vi "programa_main.vi"() -> ()   [LabVIEW 2017]
uses:
  ble_toolkit_source/type_def/connection_status_bundle.ctl
  ble_toolkit_source/type_def/address_type.ctl
  <vilib>/Platform/TimedLoop/XDataNode/timing_clust.ctl
  <vilib>/Platform/TimedLoop/XDataNode/nitl_modes.ctl
  <vilib>/Platform/TimedLoop/XDataNode/wakeup.ctl
  <vilib>/Instr/_visa.llb/VISA Configure Serial Port (Instr).vi
  <vilib>/platform/TimedLoop/XDataNode/XDataNode.xnode
  <vilib>/Platform/TimedLoop/XDataNode/XDNodeRunTimeDep.lvlib
panel:
  out "Energia consumida (mA·h)":dbl
  in  "Automàtic":bool
  in  "Manual":bool
  out "READY":bool
  in  "No Rebre Corrent":bool
  in  "Rebre Corrent":bool
  in  "No Rebre Voltatge Placa":bool
  in  "Rebre Placa":bool
  in  "No Rebre Posició":bool
  in  "Rebre Posició":bool
  in  "VISA resource name":refnum<visa-resource-name>="COM1"
  out "MAC Adrdress Seleccionada":string
  in  "MAC Address":T1=1 items=["Rueda", "Nelia"]
  out "Nom del dispsitiu conectat":string
  out "Handle table 2":string[][](array[string])
  out "Scanning":bool
  in  "Address Type":T1=1 items=["Public", "Random"]
  in  "COM Bluegiga in":refnum<visa-resource-name>="COM13"
  out "Devices":string[][](array[string])
  out "BLED112 Dongle Info":string
  out "nom fitxer":string
  out "Lectura":string
  out "Posició (º)":dbl
  out "Intensitat (mA)":dbl
  in  "?":bool
  out "Waveform Chart":dynamicdata(graph)
  out "Volatatge (V)":dbl
  out "Connection Status":T2={"MAC Address"="", "cnx handle"=0, "cnx flags"=0, "Address Type"=125, "Connection Interval (ms)"=125, "Timeout(ms)"=125, "Latency"=0, "bonding handle"=0} {"Address Type" items=["Public", "Random"]}
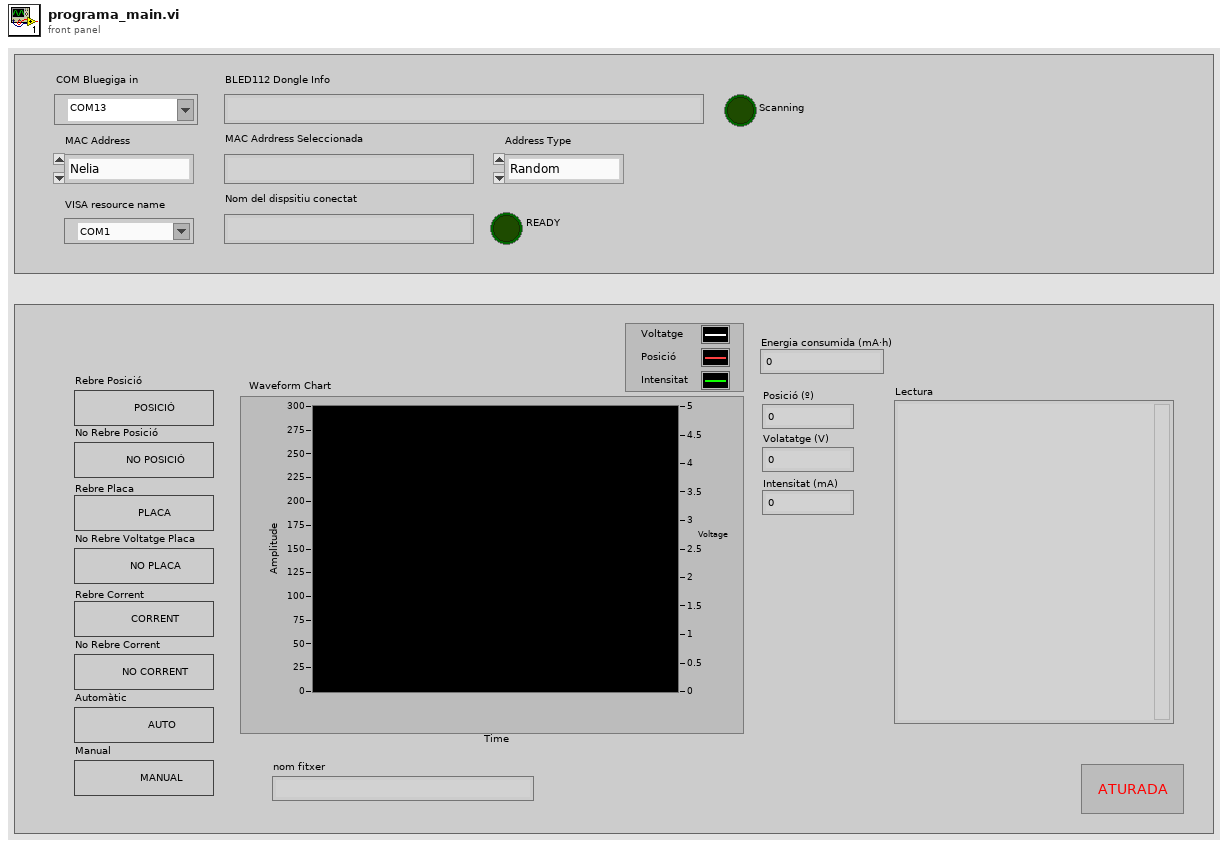
[diagram p1: front panel]
types:
  T1 = typedef "address_type.ctl" = u8
  T2 = typedef "connection_status_bundle.ctl" = cluster{"MAC Address":string, "cnx handle":u8, "cnx flags":u8, "Address Type":T1, "Connection Interval (ms)":u16, "Timeout(ms)":u16, "Latency":u16, "bonding handle":u8}
  T3 = typedef "XDNodeRunTimeDep.lvlib/timing_clust.ctl" = cluster{"Expected End [f-1]":u64, "Actual End [f-1]":u64, "Finished Late? [f-1]":bool, "Expected End [i-1]":u64, "Actual End [i-1]":u64, "Finished Late? [i-1]":bool, "Expected Start [i]":u64, "Actual Start [i]":u64, "Expected Start [f]":u64, "Actual Start [f]":u64, "Source Name":string, "Structure Name":string, "Period":i64, "Deadline":i64, "Offset":i64, "Start":i64, "Priority":i32, "Timeout":i32, "Mode":T4, "Wakeup Reason":T5, "Error":errorcluster, "Source Type":string, "Secondary Source Type":string, "Global End Time":u64, "Global Start Time":u64, "Frame Duration":u64, "Iteration Duration":u64, "Assigned CPU":i32, "I/O Scan Engine Mode":u32}
  T4 = typedef "XDNodeRunTimeDep.lvlib/nitl_modes.ctl" = enum32{"No Change", "Process missed periods, maintain original phase", "Discard missed periods, maintain original phase", "Process missed periods, ignore original phase", "Discard missed periods, ignore original phase"}
  T5 = typedef "XDNodeRunTimeDep.lvlib/wakeup.ctl" = enum32{"Normal", "Aborted", "Asynchronous wakeup", "Timing source error", "Timed loop error", "Timeout"}
  T6 = typedef "LVDateTimeRec.ctl" = cluster{"fractional second":dbl, "second":i32, "minute":i32, "hour":i32, "day of month":i32, "month":i32, "year":i32, "day of week":i32, "day of year":i32, "DST":i32}
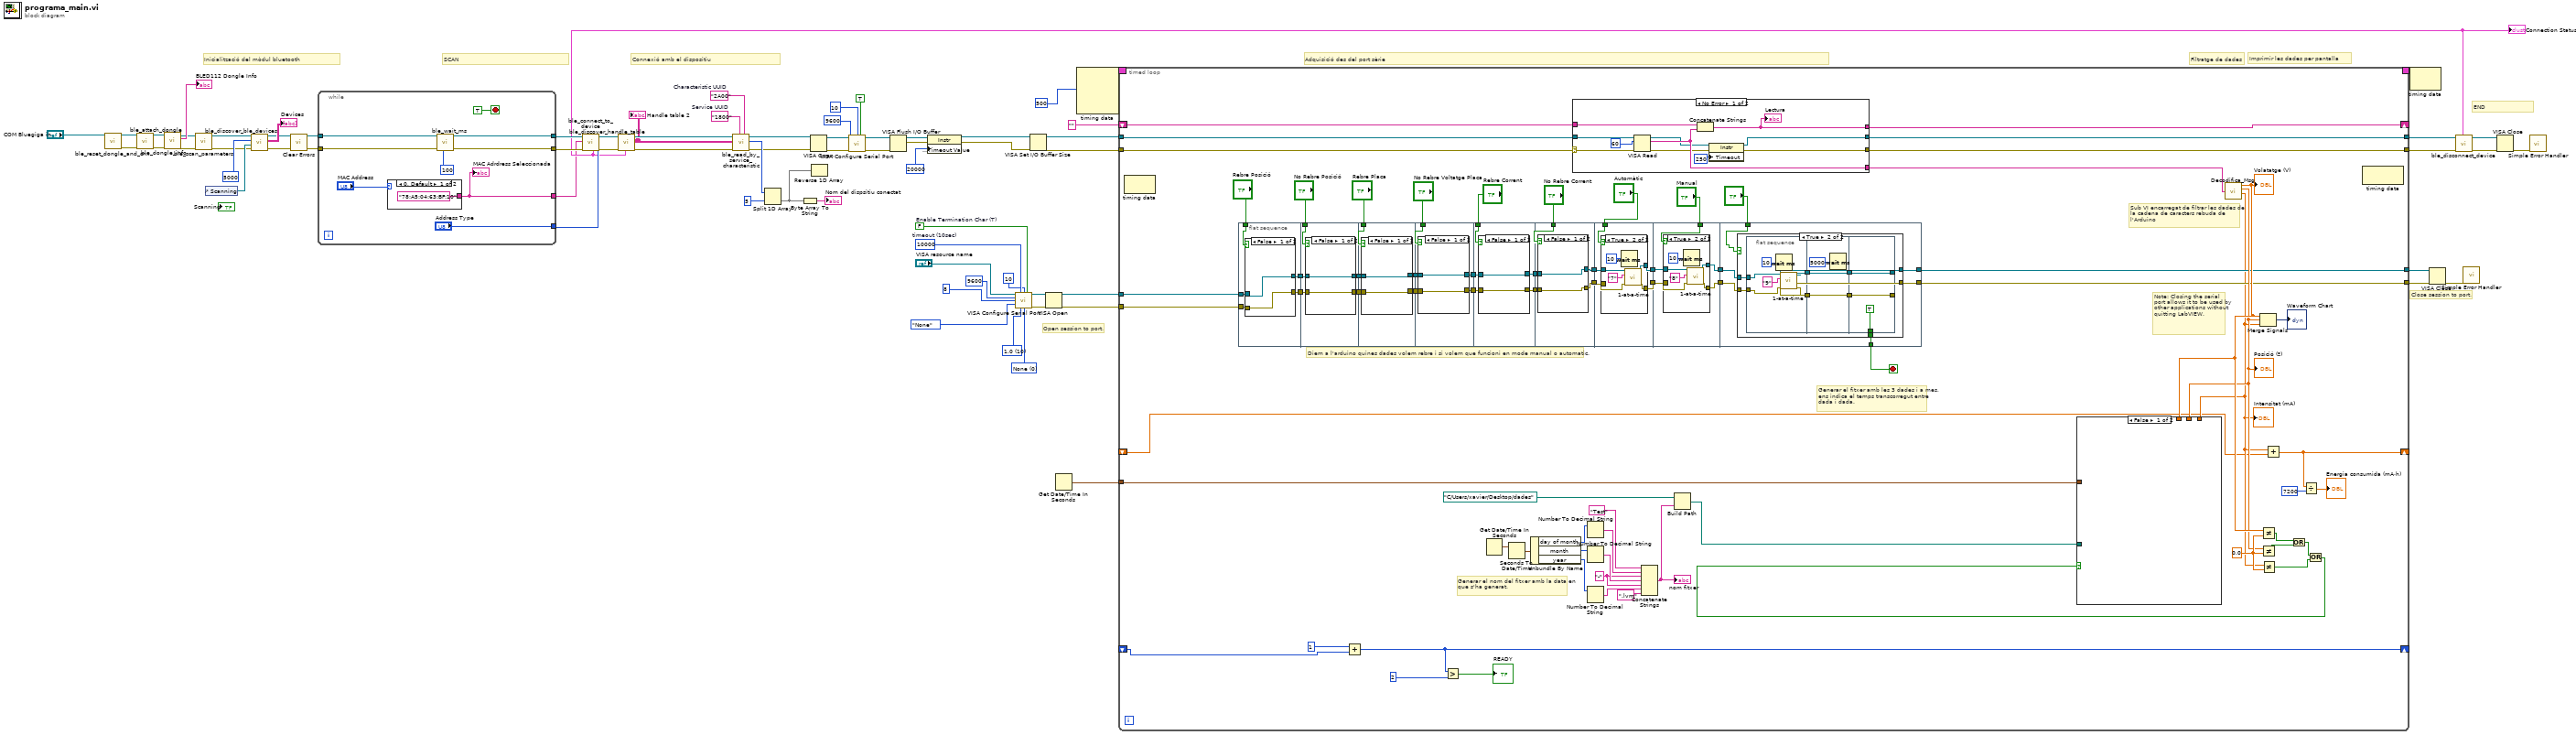
[diagram p0: block diagram]
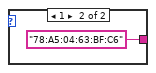
[diagram p2: hidden frame]
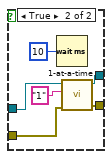
[diagram p3: hidden frame]
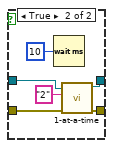
[diagram p4: hidden frame]
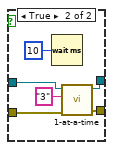
[diagram p5: hidden frame]
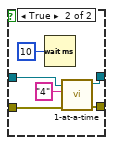
[diagram p6: hidden frame]
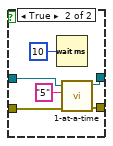
[diagram p7: hidden frame]
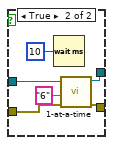
[diagram p8: hidden frame]
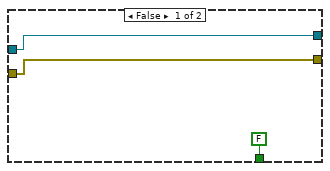
[diagram p11: hidden frame]
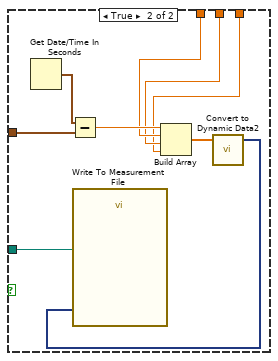
[diagram p12: hidden frame]
diagram:
  w5 = u16 0 items=["None", "XON/XOFF", "RTS/CTS", "XON/XOFF & RTS/CTS", "DTR/DSR", "XON/XOFF & DTR/DSR"] ("flow control (0:none)")
  w6 = u16 10 items=["1.0"=10, "1.5"=15, "2.0"=20] ("stop bits (10: 1 bit)")
  w17 = FALSE  # Enable Termination Char (T)
  w16 = u32 10000  # timeout (10sec)
  w32 = "2A00"  # Characteristic UUID
  w33 = "1800"  # Service UUID
  # "Open session to port."
  # "Close session to port."
  # "Imprimir les dades per pantalla"
  # "Filtratge de dades"
  # "Adquisició des del port sèrie"
  # "Connexió amb el dispositiu"
  # "SCAN"
  # "END"
  # "Inicialització del mòdul bluetooth"
  n1 = call "ble_reset_dongle_and_cnx.vi"("COM Bluegiga in"="COM Bluegiga in") -> ("error out"=w51:errorcluster, "COM Bluegiga out"=w49:refnum<visa-resource-name>)  [unwired: 9 in]
  n2 = call "ble_attach_dongle.vi"("error in (no error)"=w51, "COM Bluegiga in"=w49) -> ("error out"=w53:errorcluster, "COM Bluegiga out"=w52:refnum<visa-resource-name>)  [unwired: 8 in]
  n3 = call "ble_dongle_info.vi"("error in (no error)"=w53, "COM Bluegiga in"=w52) -> ("error out"=w56:errorcluster, "info"=→"BLED112 Dongle Info":string, "COM Bluegiga out"=w57:refnum<visa-resource-name>)  [unwired: 7 in]
  n4 = call "ble_scan_parameters.vi"("error in (no error)"=w56, "COM Bluegiga in"=w57) -> ("error out"=w54:errorcluster, "COM Bluegiga out"=w55:refnum<visa-resource-name>)  [unwired: 7 in, 1 out]
  n5 = control-ref of="Scanning"() -> (w60:refnum<vi>)
  n6 = call "ble_discover_ble_devices.vi"("error in (no error)"=w54, "LED ref"=w60, "Scan Duration (10000ms)"=u32 5000, "COM Bluegiga in"=w55) -> ("error out"=w48:errorcluster, "Devices"=→"Devices":string[][], "COM Bluegiga out"=w61:refnum<visa-resource-name>)  [unwired: 5 in]
  n7 = call <vilib>:"Clear Errors.vi"("error in (no error)"=w48) -> ("error out"=w47:errorcluster)  [unwired: 5 in, 1 out]
  n8 = while {
    tunnel: w47 -> [w82]
    tunnel: [w81] -> w59
    tunnel: w61 -> [w81]
    tunnel: [w80] -> w58
    tunnel: ["Address Type"] -> w46
    tunnel: [w76] -> w21
    stop <- TRUE stop-if-true
    n9 = case shown="0, Default" "MAC Address" {
      tunnel: ["78:A5:04:63:BF:10" "78:A5:04:63:BF:C6"] -> w76
      frame 0, Default {
      }
      frame 1 {
      }
    }
    "MAC Adrdress Seleccionada" <- w76
    n10 = call "ble_wait_ms.vi"("milliseconds to wait (100)"=u32 100, "error in (no error)"=w82) -> ("error out"=w80:errorcluster)  [unwired: 9 in]
  }
  n11 = call "ble_connect_to_device.vi"("Address Type"=w46, "error in (no error)"=w58, "MAC Address"=w21, "COM Bluegiga in"=w59) -> ("error out"=w27:errorcluster, "COM Bluegiga out"=w28:refnum<visa-resource-name>, "Connection Status"=w22:T2)  [unwired: 5 in]
  "Connection Status" <- w22
  n12 = call "ble_discover_handle_table.vi"("Connection Status"=w22, "error in (no error)"=w27, "COM Bluegiga in"=w28) -> ("error out"=w37:errorcluster, "Handle table"=w31:string[][], "COM Bluegiga out"=w36:refnum<visa-resource-name>)  [unwired: 6 in]
  "Handle table 2" <- w31
  n13 = call "ble_read_by_service_characteristic.vi"("Characteristic UUID"=w32, "Service UUID"=w33, "error in (no error)"=w37, "Handle table"=w31, "COM Bluegiga in"=w36) -> ("error out"=w25:errorcluster, "characteristic value"=w30:u8[], "COM Bluegiga out"=w26:refnum<visa-resource-name>)  [unwired: 4 in]
  n14 = Split 1D Array(array=w30, index=5) -> (second subarray=w29:u8[])  [unwired: 1 out]
  n15 = Byte Array To String(unsigned byte array=w29) -> (string=→"Nom del dispsitiu conectat":string)
  n16 = VISA Open(error in (no error)=w25, VISA resource name=w26) -> (VISA resource name=w45:refnum<visa-resource-name>, error out=w24:errorcluster)  [unwired: 3 in]
  n17 = Reverse 1D Array(array=w29) -> ()  [unwired: 1 out]
  n18 = call-poly "VISA Configure Serial Port"("VISA resource name"=w45, "termination char\n(0xA = '\\n' = LF)"=u8 10 ("termination char\n(0xA = '\\n' = LF)"), "Enable Termination\nChar (T)"=TRUE ("Enable Termination\nChar (T)"), "baud rate (9600)"=u32 9600, "error in (no error)"=w24) -> ("VISA resource name out"=w42:refnum<visa-resource-name>, "error out"=w23:errorcluster)  [unwired: 9 in]
  n19 = VISA Flush I/O Buffer(VISA resource name=w42, error in (no error)=w23) -> (VISA resource name out=w40:refnum<visa-resource-name>, error out=w39:errorcluster)  [unwired: 1 in]
  n20 = property class="Instr"(reference=w40, error in=w39, "General Settings:Timeout Value"=u32 20000) -> (reference out=w2:refnum<visa-resource-name>, error out=w1:errorcluster)
  n21 = call-poly "VISA Configure Serial Port"("VISA resource name"="VISA resource name", "timeout (10sec)"=w16, "termination char\n(0xA = '\\n' = LF)"=u8 10 ("termination char\n(0xA = '\\n' = LF)"), "Enable Termination\nChar (T)"=w17, "baud rate (9600)"=u32 9600, "data bits (8)"=u16 8, "parity (0:none)"=enum16{"None", "Odd", "Even", "Mark", "Space"}."None", "stop bits (10: 1 bit)"=w6, "flow control (0:none)"=w5) -> ("VISA resource name out"=w18:refnum<visa-resource-name>, "error out"=w19:errorcluster)  [unwired: 5 in]
  n22 = VISA Set I/O Buffer Size(VISA resource name=w2, error in (no error)=w1) -> (VISA resource name out=w4:refnum<visa-resource-name>, error out=w3:errorcluster)  [unwired: 2 in]
  n23 = VISA Open(error in (no error)=w19, VISA resource name=w18) -> (VISA resource name=w14:refnum<visa-resource-name>, error out=w13:errorcluster)  [unwired: 3 in]
  n24 = Get Date/Time In Seconds() -> (seconds since 1Jan1904=w65:timestamp)
  n25 = node-c288(i64 500 ("Period")) -> (w68:T3)  [unwired: 3 in]
  n26 = timed-loop {
    tunnel: w4 -> [w125]
    tunnel: w3 -> [w126]
    shift-right: [w153] -> _
    shift-left: "" ("read buffer") -> [w155]
    tunnel: [w152] -> w69
    tunnel: [w151] -> w70
    timing: w68 -> [_]
    timing-out: [_] -> w67
    tunnel: w65 -> [w129]
    tunnel: w14 -> [w118]
    tunnel: w13 -> [w105]
    tunnel: [w112] -> w12
    tunnel: [w111] -> w11
    shift-right: [w102] -> _
    shift-left: _ -> [w103]
    shift-right: [w89] -> _
    shift-left: _ -> [w92]
    stop <- w85 stop-if-true
    w130 = 0.0
    w142 = "-" ("string")
    # "Diem a l'arduino quines dades volem rebre i si volem que funcioni en mode manual o automatic."
    # "Generar el fitxer amb les 3 dades i a mes, ens indica el temps transcorregut entre dada i dada."
    # "Generar el nom del fitxer amb la data en que s'ha generat."
    # "Sub VI encarregat de filtrar les dades de la cadena de caracters rebuda de l'Arduino"
    # "Note: Closing the serial port allows it to be used by other applications without\nquitting LabVIEW."
    n27 = node-c288() -> ()  [unwired: 1 in, 1 out]
    n28 = flat-sequence {
      tunnel: "Rebre Posició" -> [w160]
      tunnel: w118 -> [w159]
      tunnel: [w158] -> w117
      tunnel: [w157] -> w106
      tunnel: w105 -> [w156]
      tunnel: "No Rebre Posició" -> [w173]
      tunnel: w117 -> [w172]
      tunnel: [w171] -> w116
      tunnel: [w170] -> w107
      tunnel: w106 -> [w169]
      tunnel: "Rebre Placa" -> [w186]
      tunnel: w116 -> [w185]
      tunnel: [w184] -> w115
      tunnel: [w183] -> w108
      tunnel: w107 -> [w182]
      tunnel: "No Rebre Voltatge Placa" -> [w199]
      tunnel: w115 -> [w198]
      tunnel: [w197] -> w114
      tunnel: [w196] -> w109
      tunnel: w108 -> [w195]
      tunnel: "Rebre Corrent" -> [w212]
      tunnel: w114 -> [w211]
      tunnel: [w210] -> w113
      tunnel: [w209] -> w110
      tunnel: w109 -> [w208]
      tunnel: "No Rebre Corrent" -> [w225]
      tunnel: w113 -> [w224]
      tunnel: w110 -> [w223]
      tunnel: [w222] -> w99
      tunnel: [w221] -> w98
      tunnel: w99 -> [w236]
      tunnel: w98 -> [w238]
      tunnel: [w235] -> w97
      tunnel: [w237] -> w96
      tunnel: "Automàtic" -> [w234]
      tunnel: w97 -> [w249]
      tunnel: w96 -> [w248]
      tunnel: "Manual" -> [w251]
      tunnel: [w250] -> w88
      tunnel: [w247] -> w87
      tunnel: w88 -> [w265]
      tunnel: w87 -> [w264]
      tunnel: "?" -> [w260]
      tunnel: [w261] -> w85
      tunnel: [w263] -> w112
      tunnel: [w262] -> w111
      frame #0 {
        n29 = case shown="False" w160 {
          tunnel: w159 -> [w162 w167]
          tunnel: [w162 w166] -> w158
          tunnel: [w161 w165] -> w157
          tunnel: w156 -> [w161 w164]
          frame False {
          }
          frame True {
            n30 = Wait (ms)(milliseconds to wait=u32 10) -> ()  [unwired: 1 out]
            n31 = call "1-at-a-time.vi"("error in (no error)"=w164, "write buffer"="1", "VISA resource name"=w167) -> ("error out"=w165:errorcluster, "VISA resource name out"=w166:refnum<visa-resource-name>)  [unwired: 7 in]
          }
        }
      }
      frame #1 {
        n32 = case shown="False" w173 {
          tunnel: w172 -> [w175 w180]
          tunnel: [w175 w179] -> w171
          tunnel: [w174 w178] -> w170
          tunnel: w169 -> [w174 w177]
          frame False {
          }
          frame True {
            n33 = Wait (ms)(milliseconds to wait=u32 10) -> ()  [unwired: 1 out]
            n34 = call "1-at-a-time.vi"("error in (no error)"=w177, "write buffer"="2", "VISA resource name"=w180) -> ("error out"=w178:errorcluster, "VISA resource name out"=w179:refnum<visa-resource-name>)  [unwired: 7 in]
          }
        }
      }
      frame #2 {
        n35 = case shown="False" w186 {
          tunnel: w185 -> [w188 w193]
          tunnel: [w188 w192] -> w184
          tunnel: [w187 w191] -> w183
          tunnel: w182 -> [w187 w190]
          frame False {
          }
          frame True {
            n36 = Wait (ms)(milliseconds to wait=u32 10) -> ()  [unwired: 1 out]
            n37 = call "1-at-a-time.vi"("error in (no error)"=w190, "write buffer"="3", "VISA resource name"=w193) -> ("error out"=w191:errorcluster, "VISA resource name out"=w192:refnum<visa-resource-name>)  [unwired: 7 in]
          }
        }
      }
      frame #3 {
        n38 = case shown="False" w199 {
          tunnel: w198 -> [w201 w206]
          tunnel: [w201 w205] -> w197
          tunnel: [w200 w204] -> w196
          tunnel: w195 -> [w200 w203]
          frame False {
          }
          frame True {
            n39 = Wait (ms)(milliseconds to wait=u32 10) -> ()  [unwired: 1 out]
            n40 = call "1-at-a-time.vi"("error in (no error)"=w203, "write buffer"="4", "VISA resource name"=w206) -> ("error out"=w204:errorcluster, "VISA resource name out"=w205:refnum<visa-resource-name>)  [unwired: 7 in]
          }
        }
      }
      frame #4 {
        n41 = case shown="False" w212 {
          tunnel: w211 -> [w214 w219]
          tunnel: [w214 w218] -> w210
          tunnel: [w213 w217] -> w209
          tunnel: w208 -> [w213 w216]
          frame False {
          }
          frame True {
            n42 = Wait (ms)(milliseconds to wait=u32 10) -> ()  [unwired: 1 out]
            n43 = call "1-at-a-time.vi"("error in (no error)"=w216, "write buffer"="5", "VISA resource name"=w219) -> ("error out"=w217:errorcluster, "VISA resource name out"=w218:refnum<visa-resource-name>)  [unwired: 7 in]
          }
        }
      }
      frame #5 {
        n44 = case shown="False" w225 {
          tunnel: w224 -> [w227 w232]
          tunnel: w223 -> [w226 w231]
          tunnel: [w227 w230] -> w222
          tunnel: [w226 w229] -> w221
          frame False {
          }
          frame True {
            n45 = Wait (ms)(milliseconds to wait=u32 10) -> ()  [unwired: 1 out]
            n46 = call "1-at-a-time.vi"("error in (no error)"=w231, "write buffer"="6", "VISA resource name"=w232) -> ("error out"=w229:errorcluster, "VISA resource name out"=w230:refnum<visa-resource-name>)  [unwired: 7 in]
          }
        }
      }
      frame #6 {
        n47 = case shown="True" w234 {
          tunnel: [w240 w242] -> w237
          tunnel: [w239 w243] -> w235
          tunnel: w238 -> [w239 w244]
          tunnel: w236 -> [w240 w241]
          frame False {
          }
          frame True {
            n48 = Wait (ms)(milliseconds to wait=u32 10) -> ()  [unwired: 1 out]
            n49 = call "1-at-a-time.vi"("error in (no error)"=w244, "write buffer"="7", "VISA resource name"=w241) -> ("error out"=w243:errorcluster, "VISA resource name out"=w242:refnum<visa-resource-name>)  [unwired: 7 in]
          }
        }
      }
      frame #7 {
        n50 = case shown="True" w251 {
          tunnel: [w253 w255] -> w250
          tunnel: [w252 w256] -> w247
          tunnel: w249 -> [w252 w257]
          tunnel: w248 -> [w253 w254]
          frame False {
          }
          frame True {
            n51 = Wait (ms)(milliseconds to wait=u32 10) -> ()  [unwired: 1 out]
            n52 = call "1-at-a-time.vi"("error in (no error)"=w257, "write buffer"="8", "VISA resource name"=w254) -> ("error out"=w256:errorcluster, "VISA resource name out"=w255:refnum<visa-resource-name>)  [unwired: 7 in]
          }
        }
      }
      frame #8 {
        n53 = case shown="True" w260 {
          tunnel: w265 -> [w267 w273]
          tunnel: w264 -> [w266 w272]
          tunnel: [w267 w271] -> w263
          tunnel: [w266 w270] -> w262
          tunnel: [FALSE w269] -> w261
          frame False {
          }
          frame True {
            n54 = flat-sequence {
              tunnel: w273 -> [w281]
              tunnel: w272 -> [w280]
              tunnel: [w279] -> w277
              tunnel: [w278] -> w276
              tunnel: w277 -> [w286]
              tunnel: w276 -> [w285]
              tunnel: [w286] -> w275
              tunnel: [w285] -> w274
              tunnel: [w288] -> w270
              tunnel: [w289] -> w271
              tunnel: w275 -> [w289]
              tunnel: w274 -> [w288]
              tunnel: [TRUE] -> w269
              frame #0 {
                n55 = Wait (ms)(milliseconds to wait=u32 10) -> ()  [unwired: 1 out]
                n56 = call "1-at-a-time.vi"("error in (no error)"=w280, "write buffer"="9", "VISA resource name"=w281) -> ("error out"=w278:errorcluster, "VISA resource name out"=w279:refnum<visa-resource-name>)  [unwired: 7 in]
              }
              frame #1 {
                n57 = Wait (ms)(milliseconds to wait=u32 5000) -> ()  [unwired: 1 out]
              }
              frame #2 {
              }
            }
          }
        }
      }
    }
    n58 = Add(x=1, y=w103) -> (x+y=w102:i32)
    n59 = Greater?(x=w102, y=2) -> (0:→"READY":bool)
    n60 = Get Date/Time In Seconds() -> (seconds since 1Jan1904=w149:timestamp)
    n61 = Seconds To Date/Time(time stamp (now)=w149) -> (date time rec=w148:T6)  [unwired: 1 in]
    n62 = Unbundle By Name(w148) -> ("day of month"=w147:i32, "month"=w146:i32, "year"=w145:i32)
    n63 = case "Read bytes from port." shown="No Error" w126 {
      selector: w126 -> [w310 w314]
      tunnel: [w301 w314] -> w151
      tunnel: [w302 w312] -> w152
      tunnel: [w308 _] -> w154
      tunnel: w155 -> [w309 w313]
      tunnel: [w307 w313] -> w153
      tunnel: w125 -> [w304 w312]
      frame No Error {
        n64 = VISA Read(VISA resource name=w304, byte count=u32 60 ("bytes to read"), error in (no error)=w310) -> (VISA resource name out=w306:refnum<visa-resource-name>, read buffer=w308:string, error out=w303:errorcluster)  [unwired: 1 out]
        n65 = Concatenate Strings(w309, w308) -> (w307:string)
        "Lectura" <- w307
        n66 = property class="Instr"(reference=w306, error in=w303, "Timeout"=u32 250 ("General Settings:Timeout Value")) -> (reference out=w302:refnum<visa-resource-name>, error out=w301:errorcluster)
      }
      frame Error {
      }
    }
    n67 = Number To Decimal String(number=w147) -> (decimal integer string=w144:string)  [unwired: 1 in]
    n68 = Number To Decimal String(number=w146) -> (decimal integer string=w143:string)  [unwired: 1 in]
    n69 = Number To Decimal String(number=w145) -> (decimal integer string=w141:string)  [unwired: 1 in]
    n70 = Concatenate Strings("Test" ("string"), w144, w142, w143, w142, w141, ".lvm" ("string")) -> (w138:string)
    "nom fitxer" <- w138
    n71 = Build Path(base path=path "C:/Users/xavier/Desktop/dades" ("Filename"), name or relative path=w138) -> (appended path=w136:path)
    n72 = call "Decodifica_Msg.vi"("Msg"=w154) -> ("Volts"=w128:dbl, "Graus"=w127:dbl, "Intensitat"=w93:dbl)  [unwired: 3 in]
    "Posició (º)" <- w127
    "Intensitat (mA)" <- w93
    "Volatatge (V)" <- w128
    n73 = Merge Signals(w128, w127, w93) -> (→"Waveform Chart":dynamicdata)
    n74 = Not Equal?(x=w128, y=w130) -> (x != y?=w135:bool)
    n75 = Not Equal?(x=w127, y=w130) -> (x != y?=w134:bool)
    n76 = Not Equal?(x=w93, y=w130) -> (x != y?=w132:bool)
    n77 = Add(x=w93, y=w92) -> (x+y=w89:dbl)
    n78 = Or(x=w135, y=w134) -> (x .or. y?=w133:bool)
    n79 = Divide(x=w89, y=7200) -> (x/y=→"Energia consumida (mA·h)":dbl)
    n80 = Or(x=w133, y=w132) -> (x .or. y?=w131:bool)
    n81 = case shown="False" w131 {
      tunnel: w136 -> [_ w298]
      tunnel: w129 -> [_ w294]
      tunnel: w128 -> [_ w293]
      tunnel: w127 -> [_ w292]
      tunnel: w93 -> [_ w291]
      frame False {
      }
      frame True {
        n82 = Get Date/Time In Seconds() -> (seconds since 1Jan1904=w297:timestamp)
        n83 = Subtract(x=w297, y=w294) -> (x-y=w296:dbl)
        n84 = Build Array ("Build Array 4")(w296, w293, w292, w291) -> (w295:dbl[])
        n85 = call "Convert to Dynamic Data2"("Array"=w295) -> ("Dynamic Data Type"=w290:dynamicdata)  [unwired: 3 in]
        n86 = call "Write To Measurement File"("Signals"=w290, "Filename"=w298) -> ()  [unwired: 15 in, 3 out]
      }
    }
    n87 = node-c288() -> ()  [unwired: 1 in, 1 out]
  }
  n88 = node-c288(w67) -> ()  [unwired: 1 out]
  n89 = VISA Close(VISA resource name=w12, error in (no error)=w11) -> (error out=w20:errorcluster)
  n90 = call "ble_disconnect_device.vi"("Connection Status"=w22, "error in (no error)"=w70, "COM Bluegiga in"=w69) -> ("error out"=w73:errorcluster, "COM Bluegiga out"=w74:refnum<visa-resource-name>)  [unwired: 7 in]
  n91 = call <vilib>:"Simple Error Handler.vi"("error in (no error)"=w20) -> ()  [unwired: 4 in, 5 out]
  n92 = VISA Close(VISA resource name=w74, error in (no error)=w73) -> (error out=w71:errorcluster)
  n93 = call <vilib>:"Simple Error Handler.vi"("error in (no error)"=w71) -> ()  [unwired: 1 in, 8 out]
